vi "ParseOutput.vi"(8 "error in (no error)":errorcluster, 10 "File content":string) -> (0 "error out":errorcluster, 1 "Mass compile output":string, 2 "Is successful?":bool)   [LabVIEW 2014, in "MassCompile.lvclass"]
uses:
  MassCompile.lvclass
  <vilib>/regexp/Match Regular Expression.xnode
panel:
  in  "regular expression":string="###[\\t \\r \\n \\s]+Bad[\\t \\r \\n \\s]+(.*?):[\\t \\r \\n \\s]+\"(.*?)\"[\\t \\r \\n \\s]+Path=\"(.*?)\"|CompileFile: error 1125"
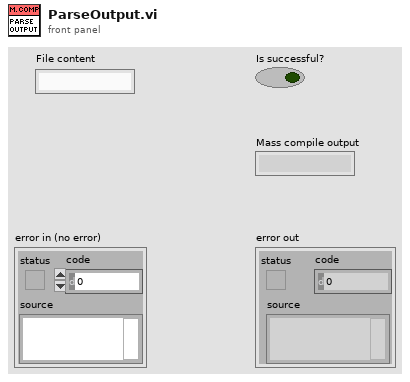
[diagram p1: front panel]
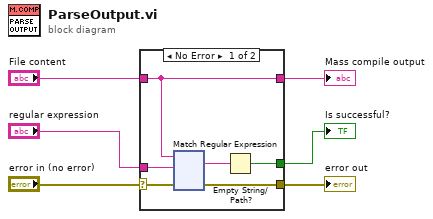
[diagram p0: block diagram]
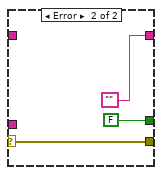
[diagram p2: hidden frame]
diagram:
  n1 = case shown="No Error" "error in (no error)" {
    selector: "error in (no error)" -> [w8 w129]
    tunnel: [w12 w129] -> w5
    tunnel: [w10 FALSE] -> w4
    tunnel: [w7 ""] -> w3
    tunnel: "regular expression" -> [w9 _]
    tunnel: "File content" -> [w7 _]
    frame No Error {
      n2 = xnode "Match Regular Expression"("input string"=w7, "regular expression"=w9, "error in"=w8) -> ("whole match"=w11:string, "error out"=w12:errorcluster)  [unwired: 3 in, 3 out]
      n3 = Empty String/Path?(string/path=w11) -> (empty?=w10:bool)
    }
    frame Error {
    }
  }
  "error out" <- w5
  "Is successful?" <- w4
  "Mass compile output" <- w3
